vi "timeWithError.vi"(3 "error in (no error)":errorcluster) -> (7 "high res \nrelative time":dbl format="%#.3f", 8 "normal time":dbl, 10 "error out":errorcluster)   [LabVIEW 2017]
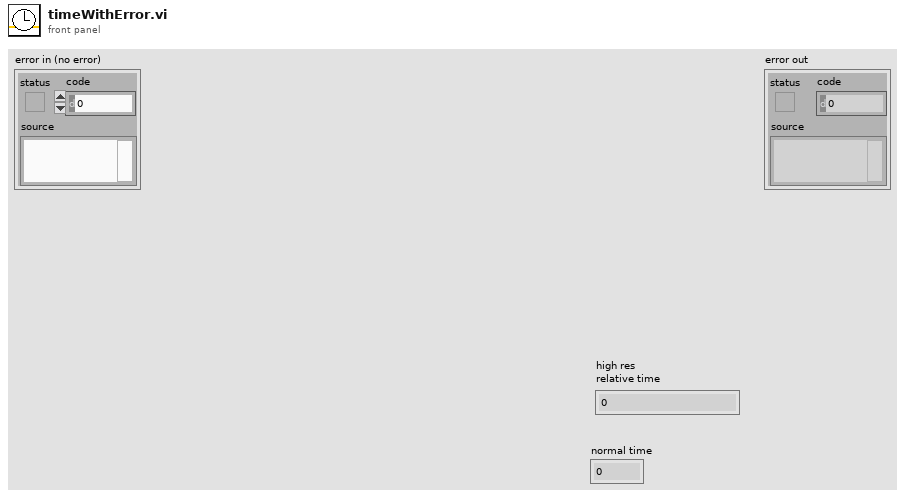
[diagram p1: front panel]
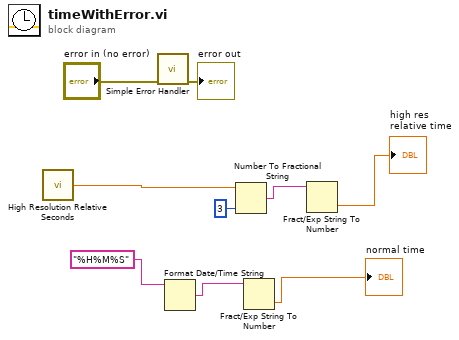
[diagram p0: block diagram]
diagram:
  n1 = call <vilib>:"High Resolution Relative Seconds.vi"() -> ("relative seconds"=w7:dbl)
  n2 = call <vilib>:"Simple Error Handler.vi"("error in (no error)"="error in (no error)") -> ("error out"=→"error out":errorcluster)  [unwired: 4 in, 4 out]
  n3 = Format Date/Time String(time format string (%c)="%H%M%S" ("time string")) -> (date/time string=w3:string)  [unwired: 2 in]
  n4 = Number To Fractional String(number=w7, precision (6)=i16 3) -> (F-format string=w5:string)  [unwired: 2 in]
  n5 = Fract/Exp String To Number(string=w3) -> (number=→"normal time":dbl)  [unwired: 3 in, 1 out]
  n6 = Fract/Exp String To Number(string=w5) -> (number=→"high res \nrelative time":dbl)  [unwired: 3 in, 1 out]
